vi "113550059隨堂測驗2.vi"() -> ()   [LabVIEW 2021]
panel:
  out "Numeric":dbl
  in  "String":string
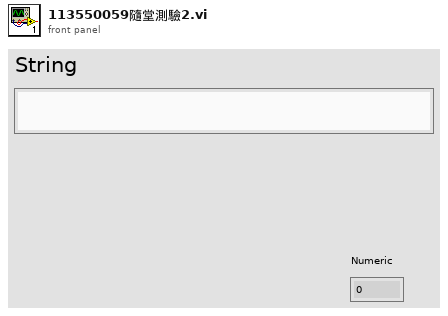
[diagram p1: front panel]
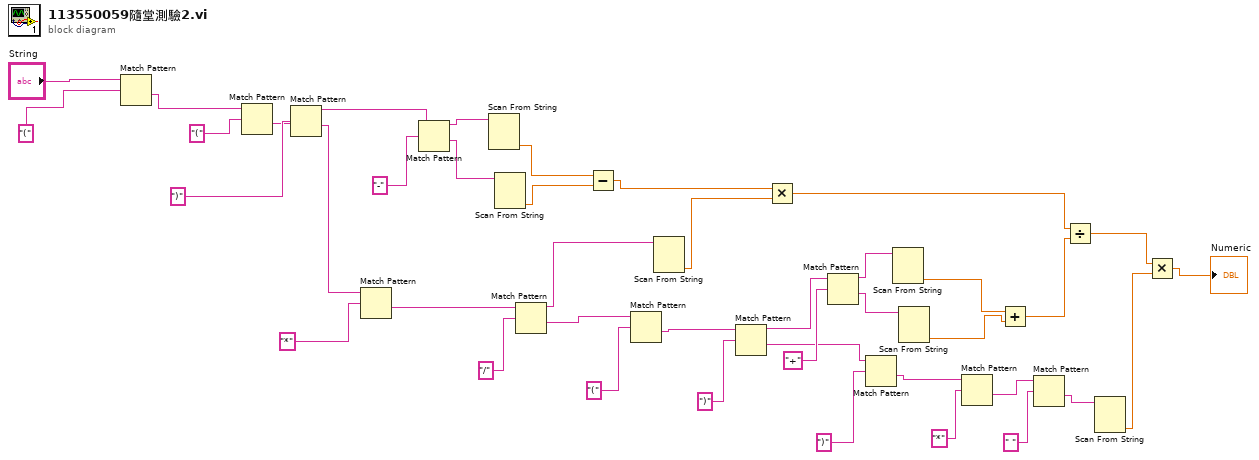
[diagram p0: block diagram]
diagram:
  n1 = Match Pattern(string="String", regular expression="(" ("search string")) -> (after substring=w39:string)  [unwired: 1 in, 3 out]
  n2 = Match Pattern(string=w39, regular expression="(" ("search string")) -> (after substring=w36:string)  [unwired: 1 in, 3 out]
  n3 = Match Pattern(string=w36, regular expression=")" ("search string")) -> (before substring=w35:string, after substring=w29:string)  [unwired: 1 in, 2 out]
  n4 = Match Pattern(string=w29, regular expression="*" ("search string")) -> (after substring=w22:string)  [unwired: 1 in, 3 out]
  n5 = Match Pattern(string=w35, regular expression="-" ("search string")) -> (before substring=w33:string, after substring=w32:string)  [unwired: 1 in, 2 out]
  n6 = Scan From String(input string=w33) -> (output 1=w30:dbl)  [unwired: 4 in, 3 out]
  n7 = Scan From String(input string=w32) -> (output 1=w31:dbl)  [unwired: 4 in, 3 out]
  n8 = Match Pattern(string=w22, regular expression="/" ("search string")) -> (before substring=w21:string, after substring=w23:string)  [unwired: 1 in, 2 out]
  n9 = Subtract(x=w30, y=w31) -> (x-y=w20:dbl)
  n10 = Match Pattern(string=w23, regular expression="(" ("search string")) -> (after substring=w18:string)  [unwired: 1 in, 3 out]
  n11 = Scan From String(input string=w21) -> (output 1=w19:dbl)  [unwired: 4 in, 3 out]
  n12 = Match Pattern(string=w18, regular expression=")" ("search string")) -> (before substring=w17:string, after substring=w11:string)  [unwired: 1 in, 2 out]
  n13 = Multiply(x=w20, y=w19) -> (x*y=w5:dbl)
  n14 = Match Pattern(string=w17, regular expression="+" ("search string")) -> (before substring=w15:string, after substring=w14:string)  [unwired: 1 in, 2 out]
  n15 = Match Pattern(string=w11, regular expression=")" ("search string")) -> (after substring=w10:string)  [unwired: 1 in, 3 out]
  n16 = Scan From String(input string=w15) -> (output 1=w13:dbl)  [unwired: 4 in, 3 out]
  n17 = Scan From String(input string=w14) -> (output 1=w12:dbl)  [unwired: 4 in, 3 out]
  n18 = Match Pattern(string=w10, regular expression="*" ("search string")) -> (after substring=w8:string)  [unwired: 1 in, 3 out]
  n19 = Add(x=w13, y=w12) -> (x+y=w4:dbl)
  n20 = Match Pattern(string=w8, regular expression=" " ("search string")) -> (after substring=w6:string)  [unwired: 1 in, 3 out]
  n21 = Divide(x=w5, y=w4) -> (x/y=w3:dbl)
  n22 = Scan From String(input string=w6) -> (output 1=w2:dbl)  [unwired: 4 in, 3 out]
  n23 = Multiply(x=w3, y=w2) -> (x*y=→"Numeric":dbl)
